vi "Get Peaks.vi"(8 "error in (no error)":errorcluster, 11 "Micron sm Digitizer in":refnum<class "Micron sm Digitizer.lvclass">) -> (0 "error out":errorcluster, 1 "Peaks per channel":i32[](array[numeric]), 2 "Peaks":dbl[](array[numeric]), 3 "Micron sm Digitizer out":refnum<class "Micron sm Digitizer.lvclass">)   [LabVIEW 2024, in "Micron sm Digitizer.lvclass"]
uses:
  Micron sm Digitizer.lvclass
  VISA Instrument/VISA Instrument.lvclass/VISA Instrument.ctl
  VISA Instrument/Read VISA resource.vi
  VISA Instrument/Write VISA resource.vi
  Micron sm Digitizer.lvclass/Micron sm Digitizer.ctl
  Micron Optics sm130/Micron Optics sm130.lvlib
panel:
  out "size(s)":i32[](array[numeric])
  out "Data Status":T1 {"Sub-Channel" items=["None", "1", "2", "3", "4"]; "Time Stamp" format="%#_20f"}
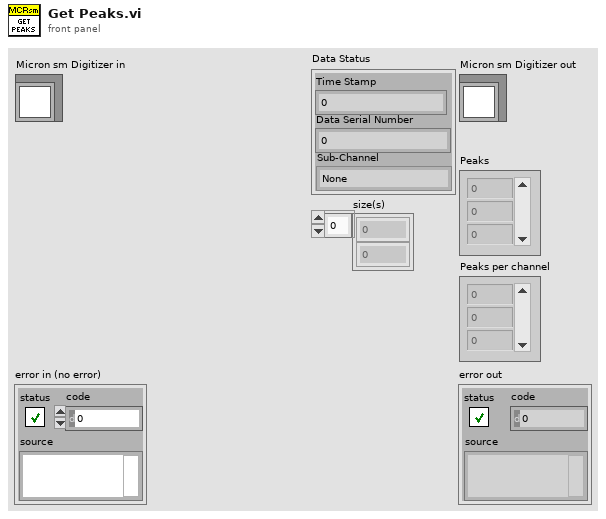
[diagram p1: front panel]
types:
  T1 = cluster{"Data Serial Number":u32, "Time Stamp":dbl, "Sub-Channel":u8}
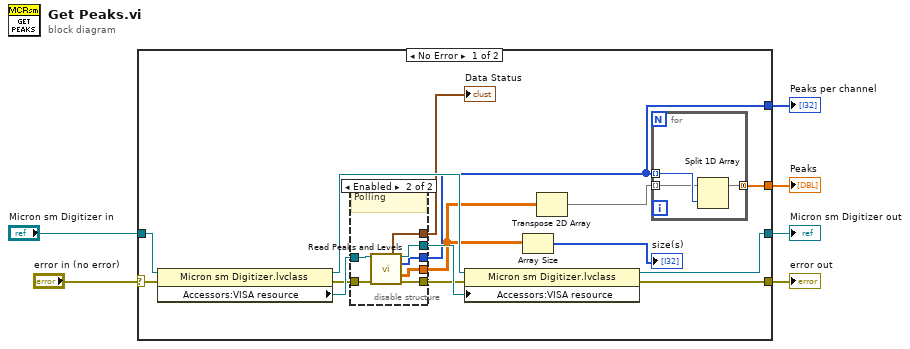
[diagram p0: block diagram]
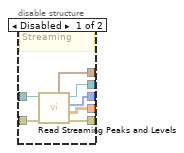
[diagram p2: hidden frame]
diagram:
  n1 = case shown="No Error" "error in (no error)" {
    selector: "error in (no error)" -> [w20 w40]
    tunnel: [w14 w40] -> w5
    tunnel: "Micron sm Digitizer in" -> [w21 w39]
    tunnel: [w13 w39] -> w3
    tunnel: [w12 _] -> w2
    tunnel: [w11 _] -> w1
    frame No Error {
      n2 = property class="Micron sm Digitizer.lvclass"(reference=w21, error in=w20) -> (reference out=w17:refnum<class "Micron sm Digitizer.lvclass">, error out=w18:errorcluster, "Accessors:VISA resource"=w19:refnum<visa-resource-name>)
      n3 = disable-structure "Diagram Disable Structure" shown="Enabled" {
        disable-tunnel: w19 -> [w28 w34]
        disable-tunnel: w18 -> [w27 w35]
        disable-tunnel: [w26 w33] -> w16
        disable-tunnel: [w25 w32] -> w15
        disable-tunnel: [w24 w30] -> w12
        disable-tunnel: [w23 w29] -> w9
        disable-tunnel: [w22 w31] -> w8
        frame Disabled {
          # "Streaming"
          n4 = call "Read Streaming Peaks and Levels.vi"("error in (no error)"=w27, "VISA resource name"=w28) -> ("error out"=w25:errorcluster, "Peak Wavelengths (nm)"=w22:dbl[][], "Number of Sensors"=w24:u16[], "VISA resource name out"=w26:refnum<visa-resource-name>, "Data Status"=w23:T1)  [unwired: 5 in]
        }
        frame Enabled {
          # "Polling"
          n5 = call "Read Peaks and Levels.vi"("VISA resource name"=w34, "error in (no error)"=w35) -> ("Data Status"=w29:T1, "VISA resource name out"=w33:refnum<visa-resource-name>, "Number of Sensors"=w30:u16[], "Peak Wavelengths (nm)"=w31:dbl[][], "error out"=w32:errorcluster)  [unwired: 5 in, 4 out]
        }
      }
      "Data Status" <- w9
      n6 = property class="Micron sm Digitizer.lvclass"(reference=w17, error in=w15, "Accessors:VISA resource"=w16) -> (reference out=w13:refnum<class "Micron sm Digitizer.lvclass">, error out=w14:errorcluster)
      n7 = Array Size(array=w8) -> (size(s)=→"size(s)":i32[])
      n8 = Transpose 2D Array(2D array=w8) -> (transposed array=w10:dbl[][])
      n9 = for {
        tunnel: w12 -> [w38] mode=indexing
        tunnel: w10 -> [w37] mode=indexing
        tunnel: [w36] -> w11 mode=concatenating
        n10 = Split 1D Array(array=w37, index=w38) -> (first subarray=w36:dbl[])  [unwired: 1 out]
      }
    }
    frame Error {
    }
  }
  "error out" <- w5
  "Micron sm Digitizer out" <- w3
  "Peaks per channel" <- w2
  "Peaks" <- w1
